vi "Cache.DUT.Write.vi"(6 "Time (now)":timestamp, 7 "Idx":i32, 8 "error in (no error)":errorcluster, 9 "Product Component":T1, 10 "Result in":T2) -> (0 "error out":errorcluster)   [LabVIEW 2016]
uses:
  Cache.TestSteps.Fglb.ResultData.ctl
  Database/ProdaNG/Controls/ProdaNG.ProcessResult.ctl
  Database/ProdaNG/Controls/ProdaNG.ProcessStepResult.ctl
  Database/ProdaNG/Controls/ProdaNG.TestStepResult.ctl
  Database/ProdaNG/Controls/ProdaNG.TestValueResult.ctl
  Database/ProdaNG/Controls/ProdaNG.ProductComponent.ctl
  Global/ApplicationGlobal.vi
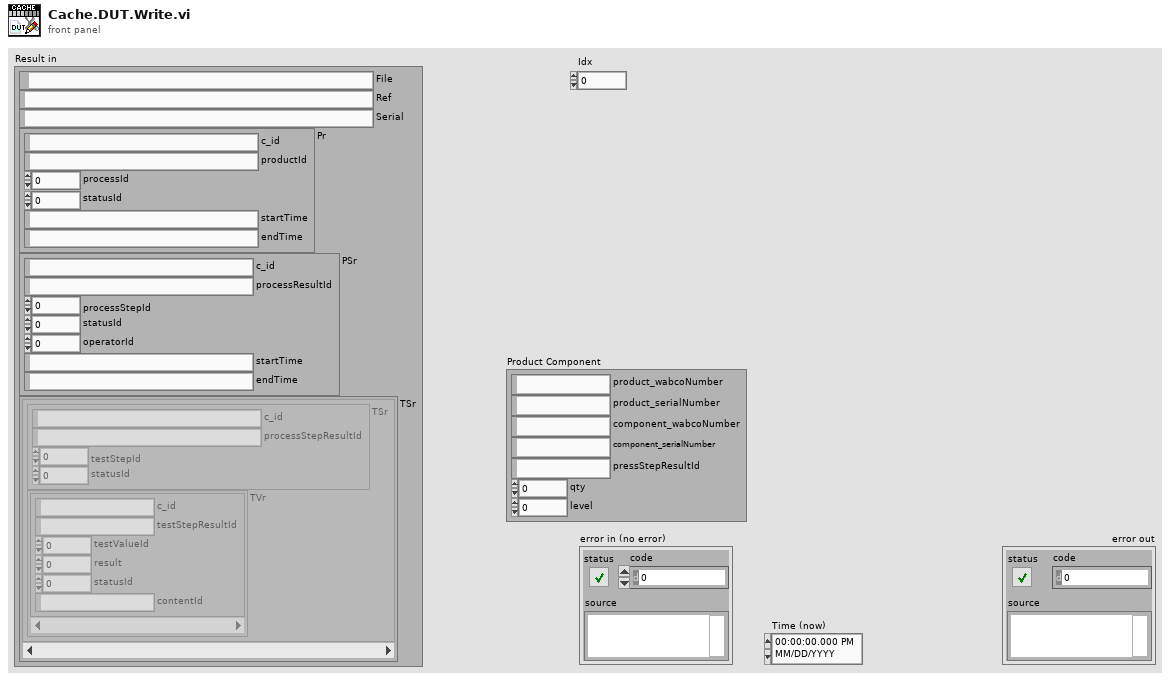
[diagram p1: front panel]
types:
  T1 = typedef "ProdaNG.ProductComponent.ctl" = cluster{"product_wabcoNumber":string, "product_serialNumber":string, "component_wabcoNumber":string, "component_serialNumber":string, "pressStepResultId":string, "qty":i32, "level":i32}
  T2 = typedef "Cache.TestSteps.Fglb.ResultData.ctl" = cluster{"File":path, "Ref":string, "Serial":string, "Pr":T3, "PSr":T4, "TSr":cluster{"TSr":T5, "TVr":T6[]}[]}
  T3 = typedef "ProdaNG.ProcessResult.ctl" = cluster{"c_id":string, "productId":string, "processId":i32, "statusId":i32, "startTime":string, "endTime":string}
  T4 = typedef "ProdaNG.ProcessStepResult.ctl" = cluster{"c_id":string, "processResultId":string, "processStepId":i32, "statusId":i32, "operatorId":i32, "startTime":string, "endTime":string}
  T5 = typedef "ProdaNG.TestStepResult.ctl" = cluster{"c_id":string, "processStepResultId":string, "testStepId":i32, "statusId":i32}
  T6 = typedef "ProdaNG.TestValueResult.ctl" = cluster{"c_id":string, "testStepResultId":string, "testValueId":i32, "result":dbl, "statusId":i32, "contentId":string}
  T7 = enum16{"open", "open or create", "create or replace", "create", "open (read-only)"}
  T8 = typedef "Cache.TestSteps.Fglb.TestData.ctl" = cluster{"Ref":string, "Desc":string, "P":T9, "PS":T10, "PP":T11[], "TS":cluster{"TS":T12, "TV":T13[], "TP":T14[]}[], "Units":T15[]}
  T9 = typedef "ProdaNG.Process.ctl" = cluster{"i_id":i32, "productionLineId":i32, "releaseId":i32, "contentId":string, "previewId":string, "mdReason":string, "mdUser":string, "mdTime":string, "description":string}
  T10 = typedef "ProdaNG.ProcessStep.ctl" = cluster{"i_id":i32, "processId":i32, "systemId":i32, "releaseId":i32, "processSequence":i32, "limitYellow":dbl, "limitRed":dbl, "mdReason":string, "mdUser":string, "mdTime":string, "filename":string, "transfer":string, "description":string}
  T11 = typedef "ProdaNG.ProcessStepParam.ctl" = cluster{"i_id":i32, "processStepId":i32, "unitId":i32, "contentId":string, "previewId":string, "value":dbl, "valueText":string, "paramSequence":i32, "history":i32, "mdReason":string, "mdUser":string, "mdTime":string, "description":string}
  T12 = typedef "ProdaNG.TestStep.ctl" = cluster{"i_id":i32, "processStepId":i32, "testSequence":i32, "testOrder":i32, "mdReason":string, "mdUser":string, "mdTime":string, "description":string}
  T13 = typedef "ProdaNG.TestValue.ctl" = cluster{"i_id":i32, "testStepId":i32, "releaseId":i32, "unitId":i32, "contentId":string, "previewId":string, "maximum":dbl, "minimum":dbl, "valueText":string, "testValueSequence":i32, "history":i32, "mdReason":string, "mdUser":string, "mdTime":string, "description":string}
  T14 = typedef "ProdaNG.TestStepParam.ctl" = cluster{"i_id":i32, "testStepId":i32, "unitId":i32, "contentId":string, "previewId":string, "value":dbl, "valueText":string, "paramSequence":i32, "history":i32, "mdReason":string, "mdUser":string, "mdTime":string, "description":string}
  T15 = typedef "ProdaNG.Unit.ctl" = cluster{"i_id":i32, "name":string, "mdReason":string, "mdUser":string, "mdTime":string, "description":string}
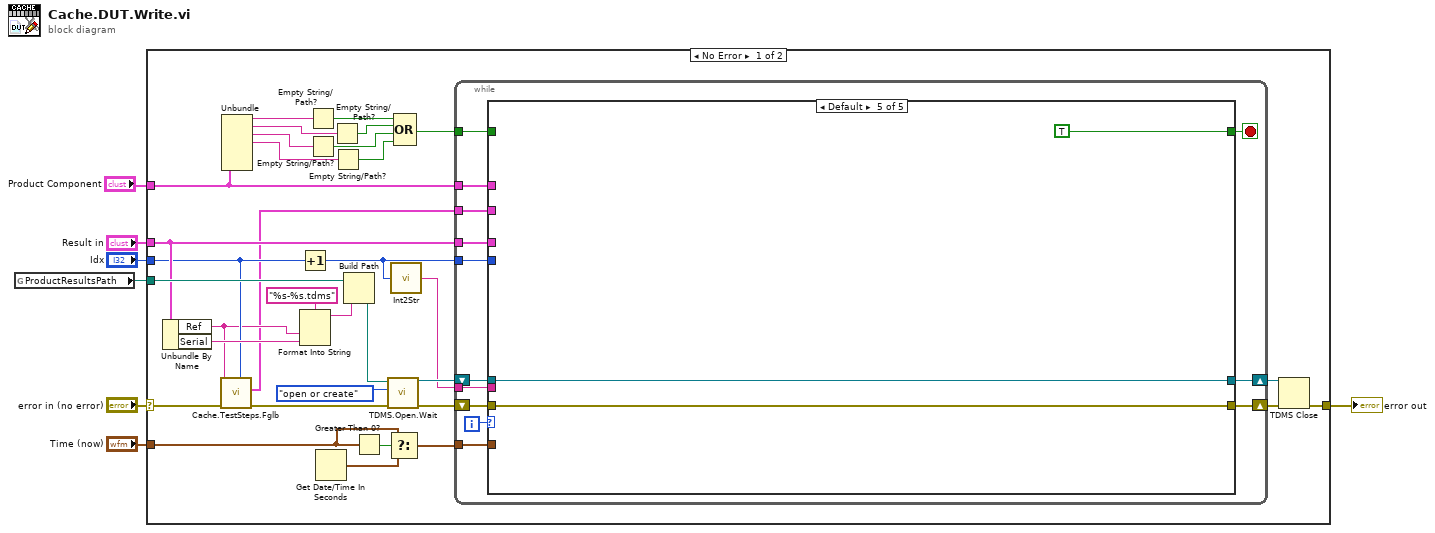
[diagram p0: block diagram]
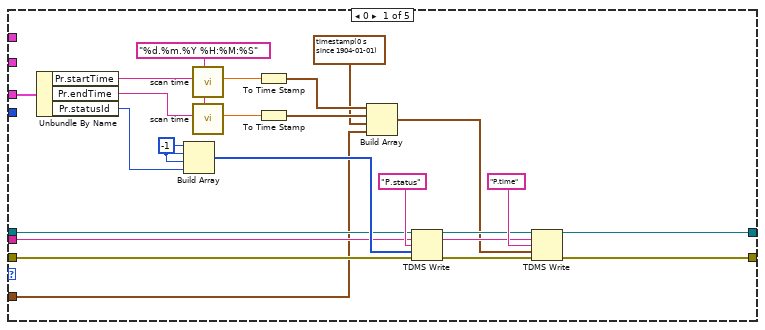
[diagram p2: hidden frame]
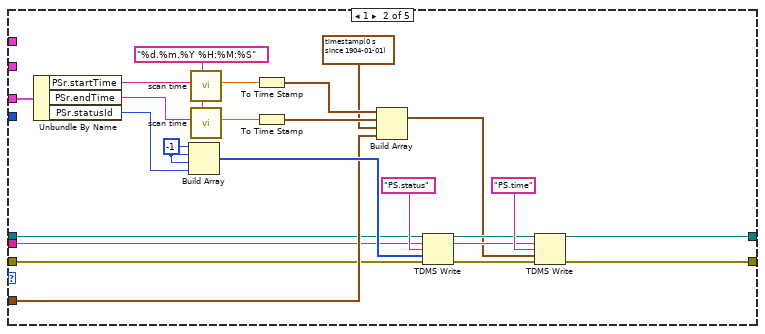
[diagram p3: hidden frame]
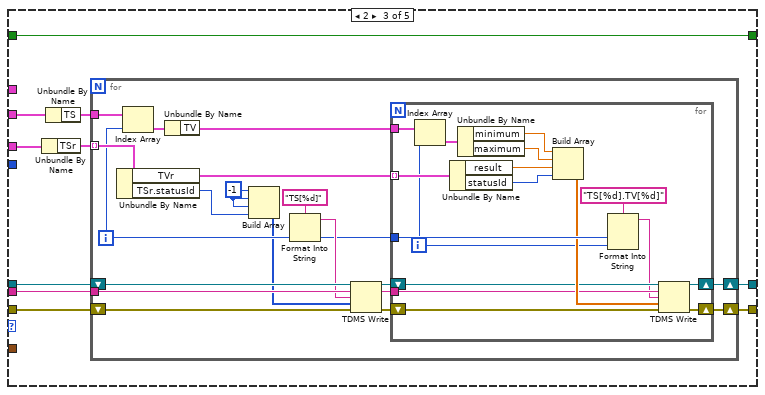
[diagram p4: hidden frame]
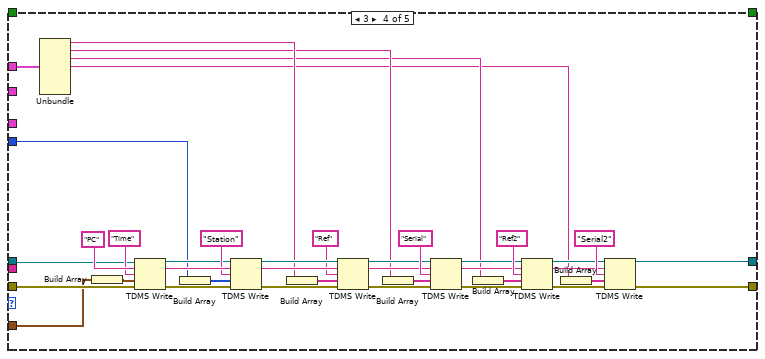
[diagram p5: hidden frame]
diagram:
  n1 = global read "ApplicationGlobal.vi" "ProductResultsPath"() -> (w4:path)
  n2 = case shown="No Error" "error in (no error)" {
    selector: "error in (no error)" -> [w25 w190]
    tunnel: "Result in" -> [w33 _]
    tunnel: [w40 w190] -> w7
    tunnel: w4 -> [w35 _]
    tunnel: "Idx" -> [w23 _]
    tunnel: "Time (now)" -> [w27 _]
    tunnel: "Product Component" -> [w13 _]
    frame No Error {
      n3 = Unbundle By Name(w33) -> ("Ref"=w22:string, "Serial"=w30:string)
      n4 = call "Cache.TestSteps.Fglb.vi"("SystemIdx"=w23, "error in (no error)"=w25, "Variant"=w22) -> ("error out"=w24:errorcluster, "Test out"=w12:T8)  [unwired: 5 in, 2 out]
      n5 = Unbundle(w13) -> ("product_wabcoNumber"=w14:string, "product_serialNumber"=w15:string, "component_wabcoNumber"=w16:string, "component_serialNumber"=w17:string)  [unwired: 3 out]
      n6 = Increment(x=w23) -> (x+1=w8:i32)
      n7 = Format Into String(format string="%s-%s.tdms" ("pattern"), w22, w30) -> (resulting string=w34:string)  [unwired: 2 in, 1 out]
      n8 = Empty String/Path?(string/path=w14) -> (empty?=w21:bool)
      n9 = Empty String/Path?(string/path=w16) -> (empty?=w19:bool)
      n10 = Get Date/Time In Seconds() -> (seconds since 1Jan1904=w29:timestamp)
      n11 = Empty String/Path?(string/path=w15) -> (empty?=w20:bool)
      n12 = Empty String/Path?(string/path=w17) -> (empty?=w18:bool)
      n13 = Build Path(base path=w35, name or relative path=w34) -> (appended path=w10:path)
      n14 = Greater Than 0?(x=w27) -> (x > 0?=w28:bool)
      n15 = call "TDMS.Open.Wait.vi"("error in (no error)"=w24, "operation (open read-only)"=T7."open or create" ("operation (0:open)"), "file path"=w10) -> ("error out"=w39:errorcluster, "tdms file out"=w31:refnum<k34>)  [unwired: 7 in]
      n16 = Select(t=w27, s=w28, f=w29) -> (s? t:f=w26:timestamp)
      n17 = call "Int2Str.vi"("Numeric"=w8) -> ("string"=w9:string)
      n18 = Compound Arithmetic op=OR(w21, w20, w19, w18) -> (w11:bool)
      n19 = while {
        tunnel: w33 -> [w49]
        shift-right: [w50] -> w38
        shift-left: w31 -> [w53]
        shift-right: [w51] -> w37
        shift-left: w39 -> [w52]
        tunnel: w9 -> [w47]
        tunnel: w12 -> [w45]
        tunnel: w26 -> [w44]
        tunnel: w8 -> [w43]
        tunnel: w13 -> [w42]
        tunnel: w11 -> [w41]
        i -> [w48]
        stop <- w46 stop-if-true
        n20 = case shown="Default" w48 {
          tunnel: w53 -> [w60 w82 w109 w157 w187]
          tunnel: w52 -> [w58 w80 w111 w158 w188]
          tunnel: [w63 w87 w110 w153 w188] -> w51
          tunnel: [w64 w88 w108 w152 w187] -> w50
          tunnel: w49 -> [w77 w101 w103 _ _]
          tunnel: w47 -> [w59 w81 w107 _ _]
          tunnel: [_ _ w102 _ TRUE] -> w46
          tunnel: w45 -> [_ _ w105 _ _]
          tunnel: w44 -> [w57 w83 _ w156 _]
          tunnel: w43 -> [_ _ _ w155 _]
          tunnel: w42 -> [_ _ _ w154 _]
          tunnel: w41 -> [_ _ w102 _ _]
          frame 0 {
            w55 = -1 ("element")
            w73 = "%d.%m.%Y %H:%M:%S" ("time format string")
            n21 = Unbundle By Name(w77) -> ("Pr.startTime"=w72:string, "Pr.endTime"=w75:string, "Pr.statusId"=w56:i32)
            n22 = Build Array(w55, w55, w55, w56) -> (w61:i32[])
            n23 = call "scan time.vi"("time format string"=w73, "formatted time string"=w72) -> ("lv time (UTC)"=w74:dbl)  [unwired: 5 in, 4 out]
            n24 = call "scan time.vi"("time format string"=w73, "formatted time string"=w75) -> ("lv time (UTC)"=w76:dbl)  [unwired: 5 in, 4 out]
            n25 = To Time Stamp(1:w74) -> (0:w70:timestamp)
            n26 = To Time Stamp(1:w76) -> (0:w69:timestamp)
            n27 = Build Array(w70, w69, timestamp(0 s since 1904-01-01) ("element"), w57) -> (w62:timestamp[])
            n28 = TDMS Write(0:w60, 5:w59, 7:"P.status", 9:w61, 11:w58) -> (4:w66:refnum<k34>, 6:w67:string, 15:w65:errorcluster)  [unwired: 1 in, 1 out]
            n29 = TDMS Write(0:w66, 5:w67, 7:"P.time", 9:w62, 11:w65) -> (4:w64:refnum<k34>, 15:w63:errorcluster)  [unwired: 1 in, 2 out]
          }
          frame 1 {
            w78 = -1 ("element")
            w97 = "%d.%m.%Y %H:%M:%S" ("time format string")
            n30 = Unbundle By Name(w101) -> ("PSr.startTime"=w96:string, "PSr.endTime"=w99:string, "PSr.statusId"=w79:i32)
            n31 = Build Array(w78, w78, w78, w79) -> (w85:i32[])
            n32 = call "scan time.vi"("time format string"=w97, "formatted time string"=w96) -> ("lv time (UTC)"=w98:dbl)  [unwired: 5 in, 4 out]
            n33 = call "scan time.vi"("time format string"=w97, "formatted time string"=w99) -> ("lv time (UTC)"=w100:dbl)  [unwired: 5 in, 4 out]
            n34 = To Time Stamp(1:w98) -> (0:w95:timestamp)
            n35 = To Time Stamp(1:w100) -> (0:w94:timestamp)
            n36 = Build Array(w95, w94, timestamp(0 s since 1904-01-01) ("element"), w83) -> (w86:timestamp[])
            n37 = TDMS Write(0:w82, 5:w81, 7:"PS.status", 9:w85, 11:w80) -> (4:w90:refnum<k34>, 6:w91:string, 15:w89:errorcluster)  [unwired: 1 in, 1 out]
            n38 = TDMS Write(0:w90, 5:w91, 7:"PS.time", 9:w86, 11:w89) -> (4:w88:refnum<k34>, 15:w87:errorcluster)  [unwired: 1 in, 2 out]
          }
          frame 2 {
            n39 = Unbundle By Name(w103) -> ("TSr"=w106:cluster{"TSr":T5, "TVr":T6[]}[])
            n40 = Unbundle By Name(w105) -> ("TS"=w104:cluster{"TS":T12, "TV":T13[], "TP":T14[]}[])
            n41 = for {
              shift-right: [w124] -> w110
              shift-left: w111 -> [w130]
              shift-right: [w121] -> w108
              shift-left: w109 -> [w129]
              tunnel: w107 -> [w128]
              tunnel: w106 -> [w119] mode=indexing
              tunnel: w104 -> [w118]
              i -> [w117]
              w112 = -1 ("element")
              n42 = Unbundle By Name(w119) -> ("TVr"=w126:T6[], "TSr.statusId"=w113:i32)
              n43 = Index Array(array=w118, index=w117) -> (element=w116:cluster{"TS":T12, "TV":T13[], "TP":T14[]})
              n44 = Unbundle By Name(w116) -> ("TV"=w115:T13[])
              n45 = Build Array(w112, w112, w112, w113) -> (w114:i32[])
              n46 = Format Into String(format string="TS[%d]", w117) -> (resulting string=w120:string)  [unwired: 2 in, 1 out]
              n47 = TDMS Write(0:w129, 5:w128, 7:w120, 9:w114, 11:w130) -> (4:w122:refnum<k34>, 6:w123:string, 15:w125:errorcluster)  [unwired: 1 in, 1 out]
              n48 = for {
                tunnel: w126 -> [w147] mode=indexing
                tunnel: w117 -> [w143]
                shift-right: [w146] -> w124
                shift-left: w125 -> [w134]
                tunnel: w123 -> [w133]
                shift-right: [w145] -> w121
                shift-left: w122 -> [w135]
                tunnel: w115 -> [w142]
                i -> [w137]
                n49 = Index Array(array=w142, index=w137) -> (element=w136:T13)
                n50 = Unbundle By Name(w147) -> ("result"=w141:dbl, "statusId"=w131:i32)
                n51 = Unbundle By Name(w136) -> ("minimum"=w138:dbl, "maximum"=w139:dbl)
                n52 = Build Array(w138, w139, w141, w131) -> (w140:dbl[])
                n53 = Format Into String(format string="TS[%d].TV[%d]", w143, w137) -> (resulting string=w132:string)  [unwired: 2 in, 1 out]
                n54 = TDMS Write(0:w135, 5:w133, 7:w132, 9:w140, 11:w134) -> (4:w145:refnum<k34>, 15:w146:errorcluster)  [unwired: 1 in, 2 out]
              }
            }
          }
          frame 3 {
            n55 = Unbundle(w154) -> ("product_wabcoNumber"=w151:string, "product_serialNumber"=w150:string, "component_wabcoNumber"=w149:string, "component_serialNumber"=w148:string)  [unwired: 3 out]
            n56 = Build Array(w156) -> (w173:timestamp[])
            n57 = TDMS Write(0:w157, 5:"PC" ("group name in (Untitled)"), 7:"Time", 9:w173, 11:w158) -> (4:w180:refnum<k34>, 6:w185:string, 15:w181:errorcluster)  [unwired: 1 in, 1 out]
            n58 = Build Array(w155) -> (w182:i32[])
            n59 = TDMS Write(0:w180, 5:w185, 7:"Station", 9:w182, 11:w181) -> (4:w184:refnum<k34>, 6:w186:string, 15:w159:errorcluster)  [unwired: 1 in, 1 out]
            n60 = Build Array(w151) -> (w160:string[])
            n61 = TDMS Write(0:w184, 5:w186, 7:"Ref", 9:w160, 11:w159) -> (4:w162:refnum<k34>, 6:w163:string, 15:w161:errorcluster)  [unwired: 1 in, 1 out]
            n62 = Build Array(w150) -> (w164:string[])
            n63 = TDMS Write(0:w162, 5:w163, 7:"Serial", 9:w164, 11:w161) -> (4:w168:refnum<k34>, 6:w167:string, 15:w166:errorcluster)  [unwired: 1 in, 1 out]
            n64 = Build Array(w149) -> (w165:string[])
            n65 = TDMS Write(0:w168, 5:w167, 7:"Ref2", 9:w165, 11:w166) -> (4:w172:refnum<k34>, 6:w175:string, 15:w171:errorcluster)  [unwired: 1 in, 1 out]
            n66 = Build Array(w148) -> (w177:string[])
            n67 = TDMS Write(0:w172, 5:w175, 7:"Serial2", 9:w177, 11:w171) -> (4:w152:refnum<k34>, 15:w153:errorcluster)  [unwired: 1 in, 2 out]
          }
          frame Default {
          }
        }
      }
      n68 = TDMS Close(8:w37, 11:w38) -> (0:w40:errorcluster)  [unwired: 1 out]
    }
    frame Error {
    }
  }
  "error out" <- w7
